vi "NewLogReader.vi"() -> ()   [LabVIEW 2011]
doc: "Reads new (11-1-2012+) style logs and displays the data in a human-understandable format."
uses:
  0-OCU/0 Typedefs/Rudder Position.ctl
  2-Think/2 Typedefs/apparent wind direction.ctl
  2-Think/2 Typedefs/apparent wind speed.ctl
  2-Think/2 Typedefs/apparent wind.ctl
  2-Think/2 Typedefs/heading.ctl
  2-Think/2 Typedefs/UTM Location.ctl
  2-Think/2 Typedefs/robot velocity.ctl
  2-Think/2 Typedefs/pitch and roll.ctl
  0-OCU/0 Typedefs/Apparent Wind Point of Sail.ctl
  0-OCU/0 Typedefs/Maps.ctl
  0-OCU/0 Typedefs/Sail Position.ctl
  2-Think/2 Typedefs/UTM Circle.ctl
  <vilib>/vision/Image Controls.llb/IMAQ Image.ctl
  2-Think/2 Classes/Waypoint/Waypoint.lvclass
panel:
  in  "Choose graph to display":T1(tab)
  out "Rudder Manual?":bool
  out "Rudder Position":T2 scale=50.0..-50.0 scale format="%#.2g"
  out "Sail Manual?":bool
  in  "OCU":enum32{"Mission Map", "Detailed Telemetry"}(tab)
  out "Heading":T3 format="%05.1f"
  out "Goodness Functions Polar Plot":picture
  in  "Plot Colors":T4={"Target"=3381759, "No Sail"=16711680, "Change"=16756736, "Pure Waypt"=35080, "Pure Wind"=16860, "Combined"=16777228}
  out "Mission Map":T5(plugin-control)
  out "Apparent Wind Direction\nPoint of Sail":T6 scale=0.0..360.0 scale format="%4d"
  in  "Font Size":i16=40
  in  "Globals":enum32{"Where Am I", "What's Around Me"}(tab)
  out "Robot Heading":T3 format="%05.1f"
  out "Robot UTM Location":T7 {"North" format="%#_10f"; "East" format="%#_8f"}
  out "Robot Velocity":T8
  out "Robot Pitch/Roll":T9 {"Roll" format="%05.1f"; "Pitch" format="%05.1f"}
  out "Robot Speed (m/s)":dbl
  out "Apparent Wind Direction":T10
  out "Apparent Wind Speed":T11
  out "Apparent Wind":T12
  in  "Map Name":T13="LPB Pool"
  out "Sail Position":T14
  out "Location":cluster{dbl[], dbl[]}[](graph)
  out "Battery Voltage":cluster{i32[], dbl[]}(graph)
  out "Velocity":cluster{i32[], dbl[]}[](graph)
  out "Headings":cluster{i32[], dbl[]}[](graph)
  out "Rudder":cluster{i32[], dbl[]}(graph)
  out "Sail":cluster{i32[], dbl[]}(graph)
  in  "Time":i32(slide) max=625 scale=0.0..42.0
  in  "stop":bool
  in  "Array":string[](array[string])=["RobotLocation", "RobotHeading", "RobotVelocity", "RobotPitch", "RobotRoll", "BatteryVoltage", "ApparentWindDirection", "ApparentWindSpeed", "Rudder", "Sail", "GoodnessFunctions", "NoSailZones", "Waypoint#", "WaypointTolerance", "WaypointCoordinates", "OverrideRudder", "OverrideSail"]
  out "Processing File....":path
  in  "Stop early":bool
  out "Percent Complete":u8(slide) scale=0.0..100.0
  # "As Measured"
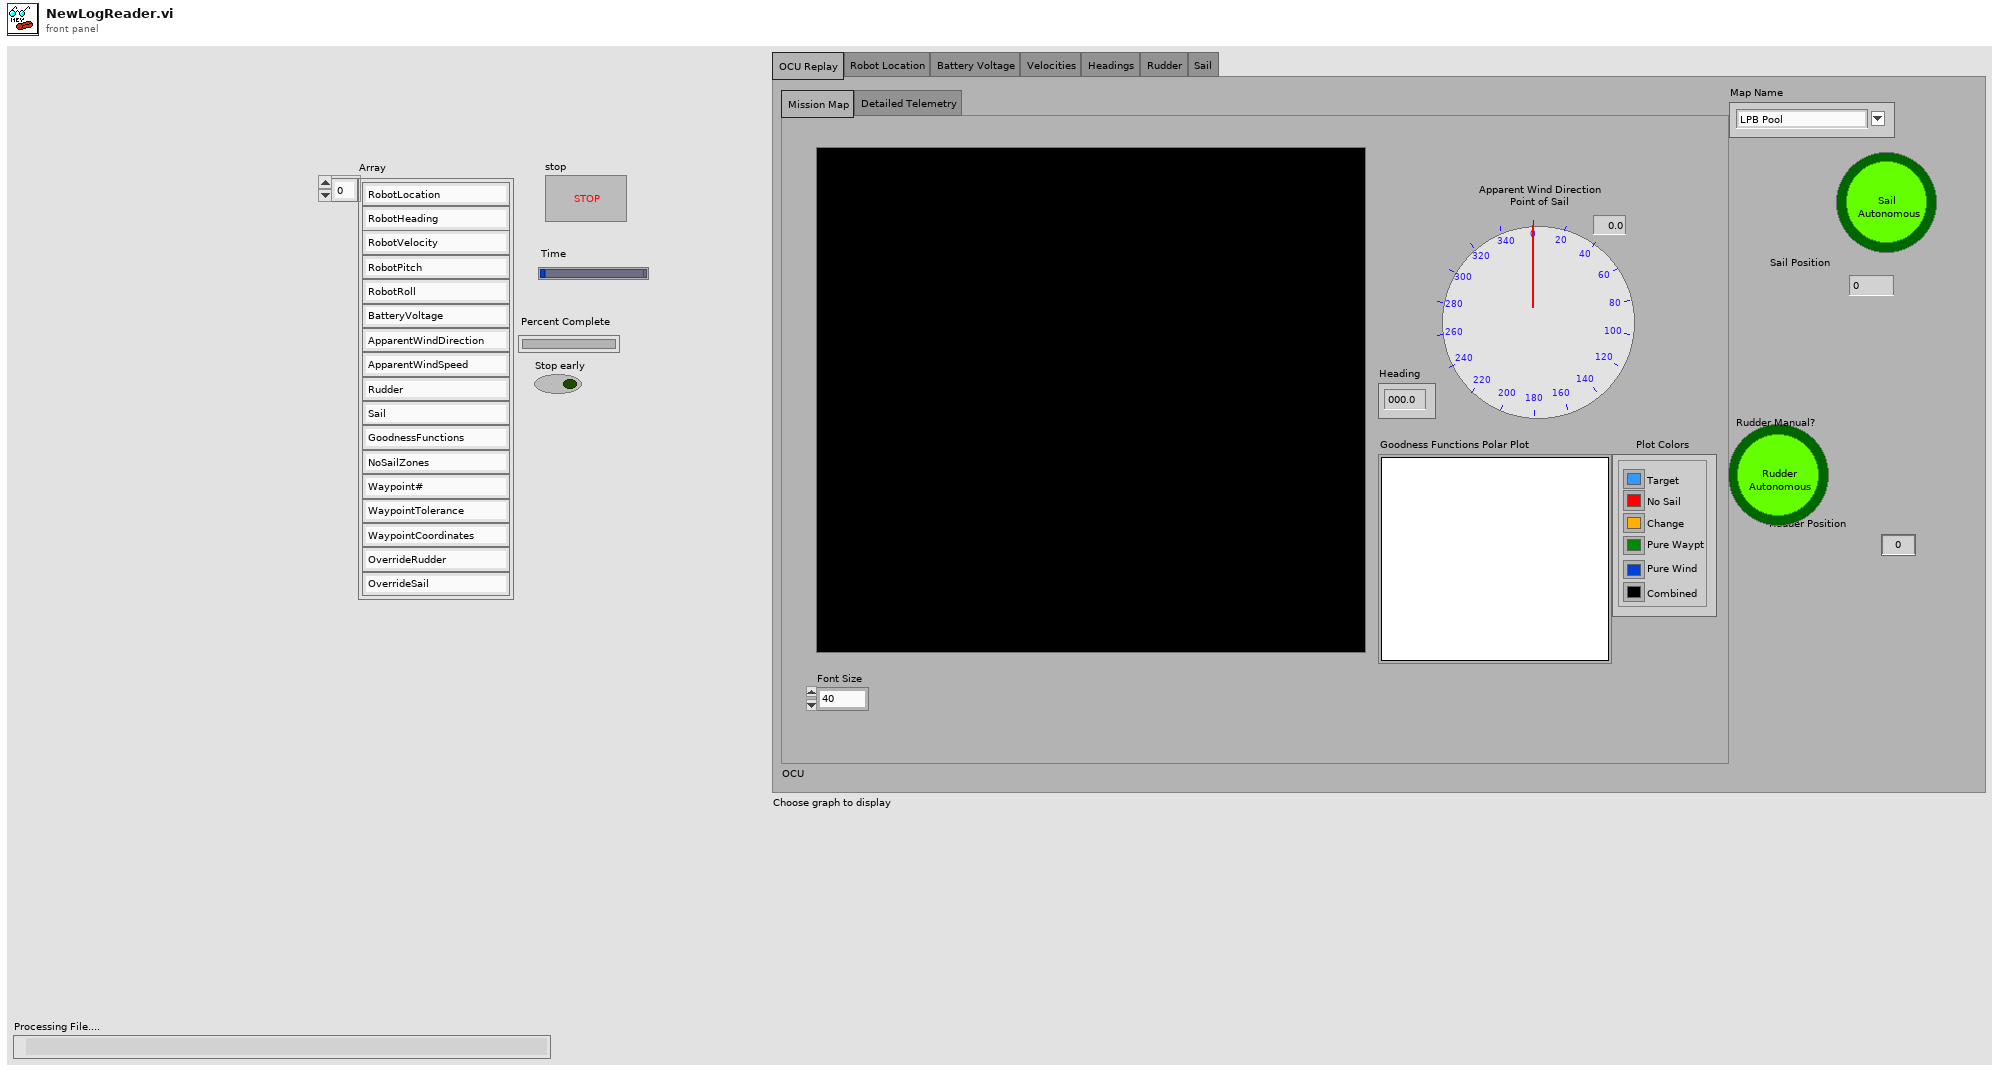
[diagram p1: front panel]
types:
  T1 = enum32{"OCU Replay", "Robot Location", "Battery Voltage", "Velocities", "Headings", "Rudder", "Sail"}
  T2 = typedef "Rudder Position.ctl" = dbl
  T3 = typedef "heading.ctl" = dbl
  T4 = cluster{"Target":u32, "No Sail":u32, "Change":u32, "Pure Waypt":u32, "Pure Wind":u32, "Combined":u32}
  T5 = typedef "IMAQ Image.ctl" = refnum<image>
  T6 = typedef "Apparent Wind Point of Sail.ctl" = dbl
  T7 = typedef "UTM Location.ctl" = cluster{"UTM Zone":dbl, "Hemisphere":enum16{"North", "South"}, "East":dbl, "North":dbl}
  T8 = typedef "robot velocity.ctl" = cluster{"East":dbl, "North":dbl}
  T9 = typedef "pitch and roll.ctl" = cluster{"Pitch":dbl, "Roll":dbl}
  T10 = typedef "apparent wind direction.ctl" = dbl
  T11 = typedef "apparent wind speed.ctl" = dbl
  T12 = typedef "apparent wind.ctl" = cluster{"Toward Fore":dbl, "Toward Starboard":dbl}
  T13 = typedef "Maps.ctl" = string
  T14 = typedef "Sail Position.ctl" = dbl
  T15 = typedef "UTM Circle.ctl" = cluster{"UTM Zone":dbl, "Hemisphere":enum16{"North", "South"}, "East":dbl, "North":dbl, "Radius":dbl}
  T16 = cluster{"RobotHeading":dbl, "RobotSpeed":dbl, "RobotPitch":dbl, "RobotRoll":dbl, "BatteryVoltage":dbl, "ApparentWindDirection":dbl, "ApparentWindSpeed":dbl, "Rudder":dbl, "Sail":dbl, "Waypoint#":dbl, "WaypointTolerance":dbl, "GoodnessFunctions":string, "OverrideRudder":bool, "OverrideSail":bool, "Global No Sail Circles":T15[], "Robot Location":T7, "WaypointCoordinates":T7}
  T17 = typedef "0-Image Descriptor.ctl" = cluster{"Upper-Left Corner Coordinates":T7, "Meters/Pixel":dbl}
  T18 = typedef "Velocity.ctl" = cluster{"East":dbl, "North":dbl}
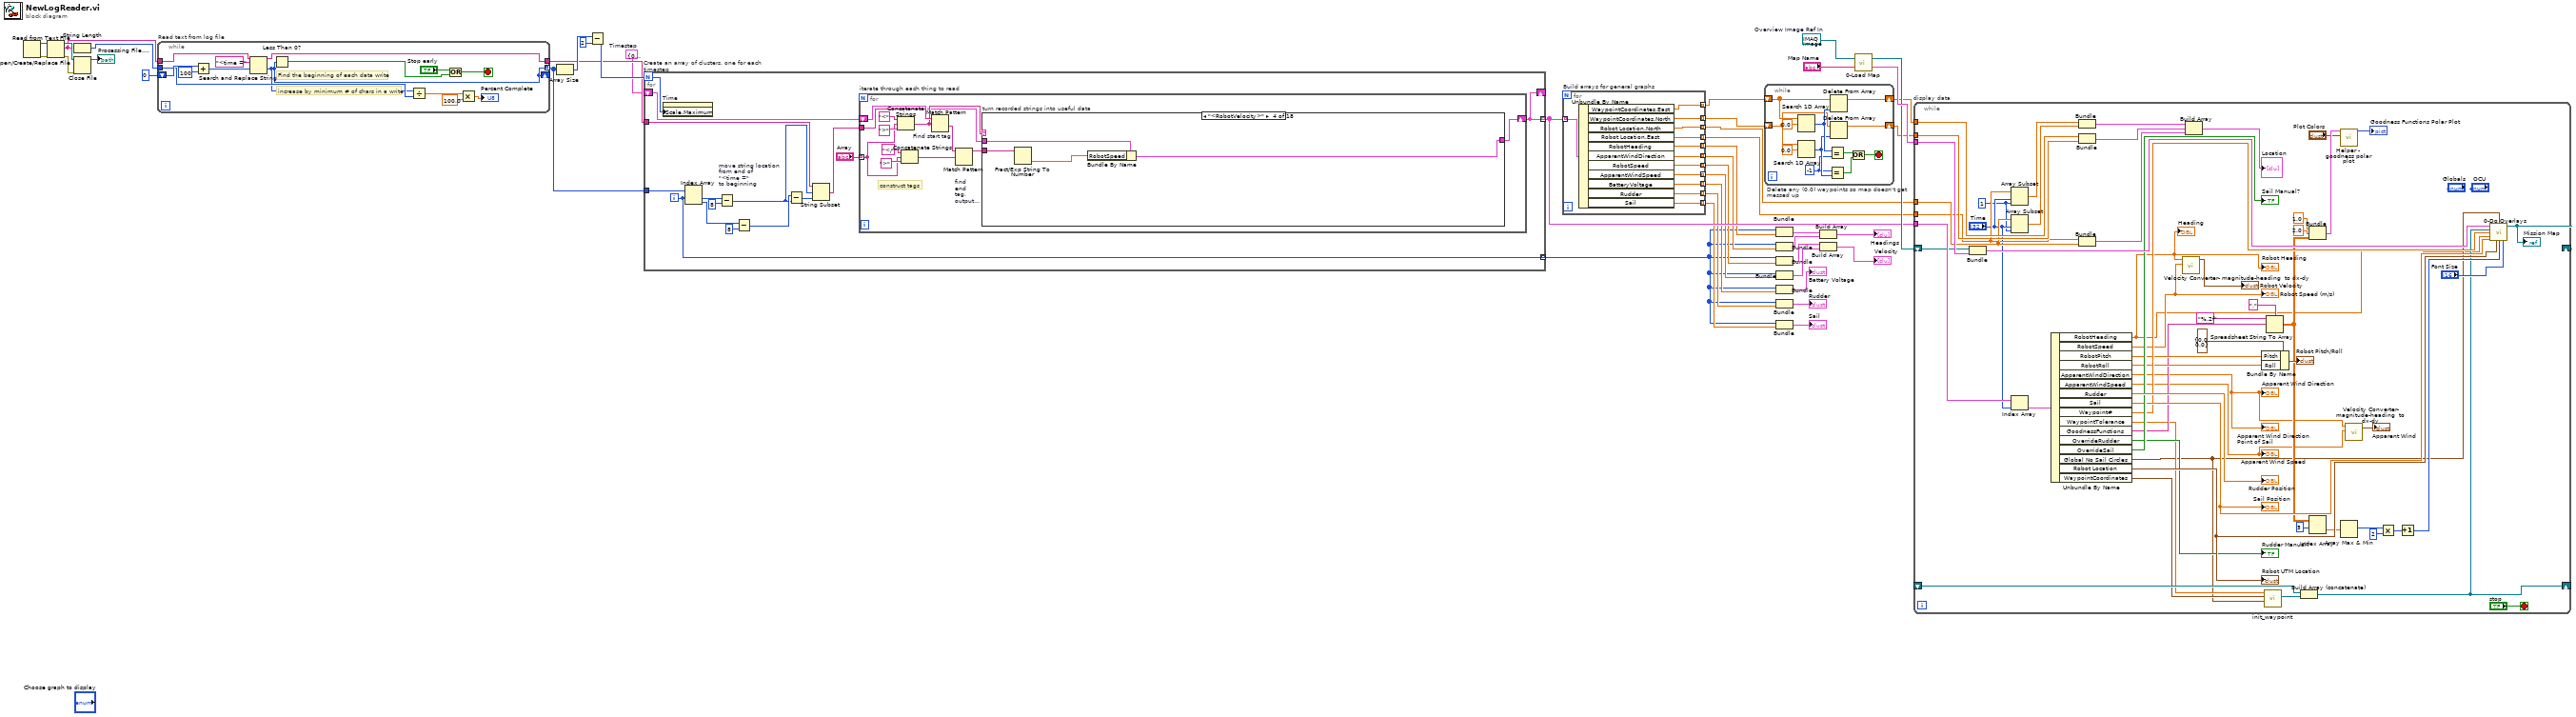
[diagram p0: block diagram]
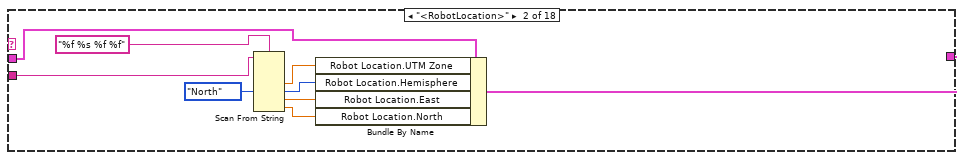
[diagram p3: hidden frame]
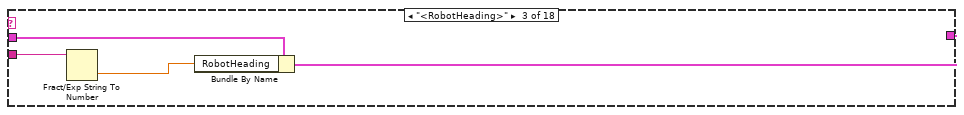
[diagram p4: hidden frame]
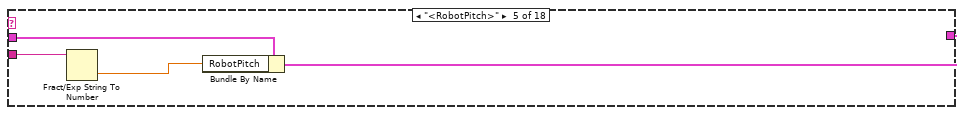
[diagram p5: hidden frame]
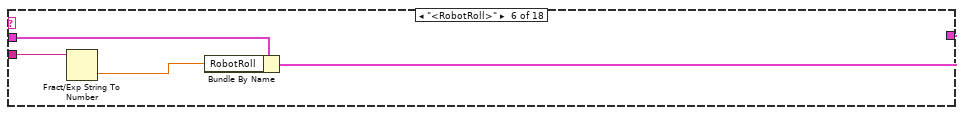
[diagram p6: hidden frame]
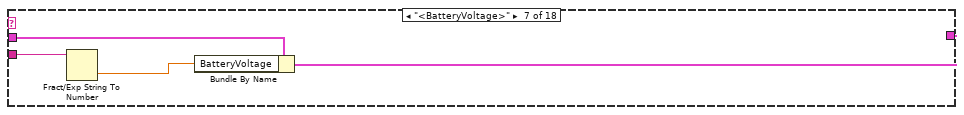
[diagram p7: hidden frame]
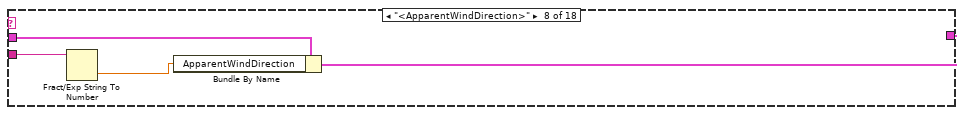
[diagram p8: hidden frame]
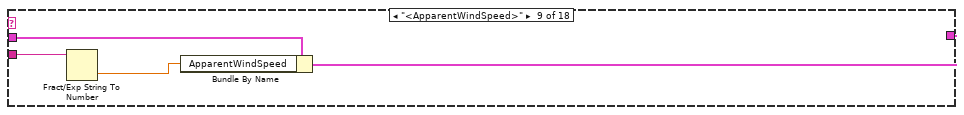
[diagram p9: hidden frame]
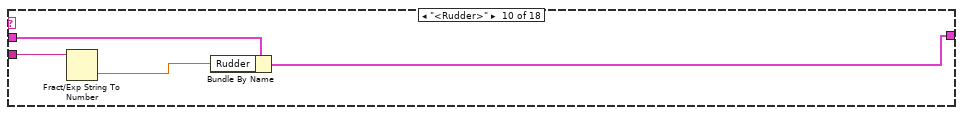
[diagram p10: hidden frame]
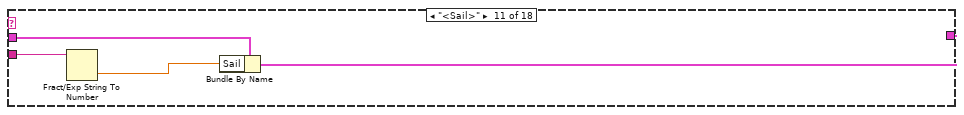
[diagram p11: hidden frame]
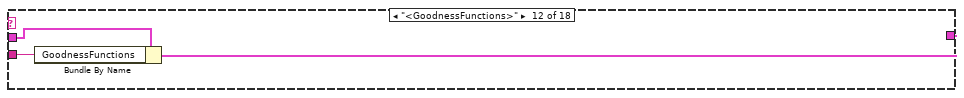
[diagram p12: hidden frame]
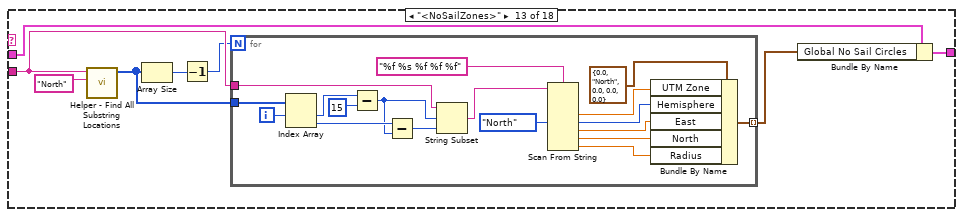
[diagram p13: hidden frame]
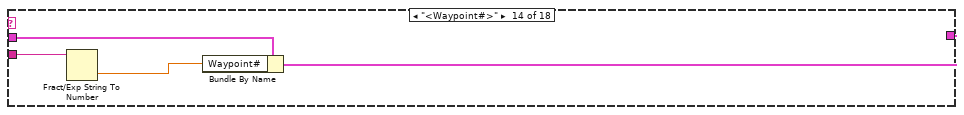
[diagram p14: hidden frame]
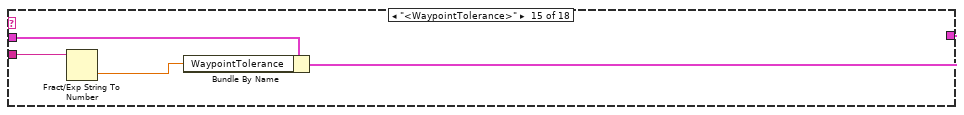
[diagram p15: hidden frame]
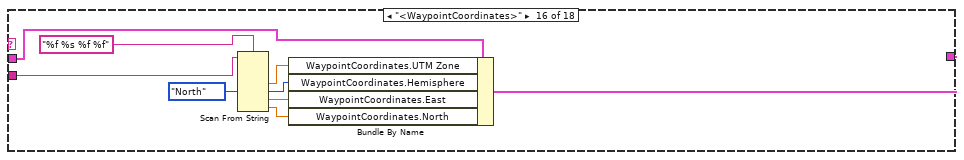
[diagram p16: hidden frame]
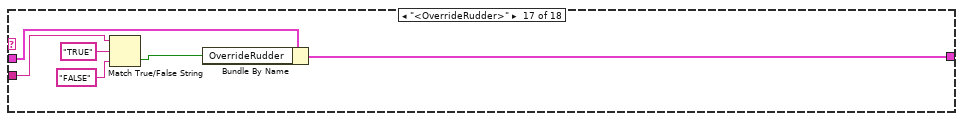
[diagram p17: hidden frame]
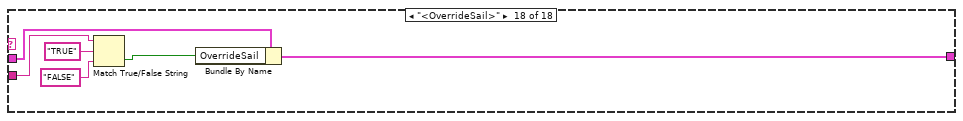
[diagram p18: hidden frame]
diagram:
  w28 = T5 refnum  # Overview Image Ref In
  w26 = T16 {"RobotHeading"=0.0, "RobotSpeed"=0.0, "RobotPitch"=0.0, "RobotRoll"=0.0, "BatteryVoltage"=0.0, "ApparentWindDirection"=0.0, "ApparentWindSpeed"=0.0, "Rudder"=0.0, "Sail"=0.0, "Waypoint#"=0.0, "WaypointTolerance"=0.0, "GoodnessFunctions"="", "OverrideRudder"=FALSE, "OverrideSail"=FALSE, "Global No Sail Circles"=[], "Robot Location"={"UTM Zone"=0.0, "Hemisphere"=enum."North", "East"=0.0, "North"=0.0}, "WaypointCoordinates"={"UTM Zone"=0.0, "Hemisphere"=enum."North", "East"=0.0, "North"=0.0}}  # Timestep
  n1 = Open/Create/Replace File() -> (refnum out=w42:refnum<file>, error out=w38:errorcluster)  [unwired: 6 in, 1 out]
  n2 = Read from Text File(file (use dialog)=w42, error in=w38) -> (refnum out=w39:refnum<file>, text=w36:string, error out=w40:errorcluster)  [unwired: 2 in, 1 out]
  n3 = String Length(string=w36) -> (length=w35:i32)
  n4 = Close File(refnum=w39, error in=w40) -> (path=→"Processing File....":path)  [unwired: 1 out]
  n5 = while "Read text from log file" {
    tunnel: w36 -> [w46]
    shift-right: [w44] -> _
    shift-left: 0 ("offset past replacement") -> [w56]
    tunnel: [w45] -> w30
    tunnel: [w44] -> w31 mode=indexing
    tunnel: w35 -> [w48]
    stop <- w54 stop-if-true
    # "increase by minimum # of chars in a write"
    # "Find the beginning of each data write"
    n6 = Add(x=w56, y=100) -> (x+y=w47:i32)
    n7 = Search and Replace String(input string=w46, search string="<time =", offset=w47) -> (result string=w45:string, offset past replacement=w44:i32)  [unwired: 5 in, 2 out]
    n8 = Less Than 0?(x=w44) -> (x < 0?=w52:bool)
    n9 = Divide(x=w44, y=w48) -> (x/y=w51:dbl)
    n10 = Or(x="Stop early", y=w52) -> (x .or. y?=w54:bool)
    n11 = Multiply(x=w51, y=100.0) -> (x*y=→"Percent Complete":dbl)
  }
  n12 = Array Size(array=w31) -> (size(s)=w34:i32)
  n13 = Subtract(x=w34, y=2) -> (x-y=w32:i32)
  n14 = for "Create an array of clusters, one for each timestep" {
    N: w32 -> [w62]
    tunnel: w31 -> [w71]
    tunnel: w30 -> [w66]
    tunnel: [w61] -> w24 mode=indexing
    shift-right: [w61] -> _
    shift-left: w26 -> [w60]
    tunnel: [w57] -> w5 mode=indexing
    i -> [w57]
    n15 = property on="Time" class="Slide (strict)"("Scale.Maximum"=w62) -> ()  [unwired: 2 in, 2 out]
    n16 = Index Array(array=w71, index #1=w57) -> (element #1=w70:i32, element #2=w67:i32)  [unwired: 1 in]
    n17 = Subtract "move string location\nfrom end of \n\"<time =\"\nto beginning"(x=w70, y=8) -> (x-y=w58:i32)
    n18 = Subtract(x=w67, y=8) -> (x-y=w59:i32)
    n19 = Subtract(x=w59, y=w58) -> (x-y=w65:i32)
    n20 = String Subset(string=w66, offset (0)=w58, length (rest)=w65) -> (substring=w64:string)
    n21 = for "iterate through each thing to read" {
      tunnel: w64 -> [w82]
      tunnel: "Array" -> [w77] mode=indexing
      shift-right: [w75] -> w61
      shift-left: w60 -> [w72]
      # "construct tags"
      n22 = Concatenate Strings("<" ("string"), w77, ">" ("string")) -> (w78:string)
      n23 = Concatenate Strings("</" ("string"), w77, ">" ("string")) -> (w79:string)
      n24 = Match Pattern "Find start tag"(string=w82, regular expression=w78) -> (after substring=w73:string)  [unwired: 1 in, 3 out]
      n25 = Match Pattern "find\nend\ntag,\noutput\nbetween\ntags"(string=w73, regular expression=w79) -> (before substring=w74:string)  [unwired: 1 in, 3 out]
      n26 = case "turn recorded strings into useful data" shown="\"<RobotVelocity>\"" w78 {
        tunnel: w74 -> [_ w87 w97 w100 w103 w108 w110 w114 w118 w122 w126 w131 w138 w160 w163 w167 w176 w182]
        tunnel: w72 -> [w84 w89 w96 w101 w104 w107 w112 w116 w120 w124 w128 w132 w137 w161 w165 w174 w179 w184]
        tunnel: [w84 w88 w94 w98 w102 w106 w111 w115 w119 w123 w127 w130 w135 w159 w164 w170 w177 w183] -> w75
        frame Default {
          # "hopefully never needs to be used"
        }
        frame "<RobotLocation>" {
          n27 = Scan From String(format string="%f %s %f %f", input string=w87, default 2=enum16{"North", "South"}."North" ("Robot Location.Hemisphere")) -> (output 1=w92:dbl, output 2=w85:enum16{"North", "South"}, output 3=w91:dbl, output 4=w90:dbl)  [unwired: 5 in, 3 out]
          n28 = Bundle By Name(cluster=w89, "Robot Location.UTM Zone"=w92, "Robot Location.Hemisphere"=w85, "Robot Location.East"=w91, "Robot Location.North"=w90) -> (w88:T16)
        }
        frame "<RobotHeading>" {
          n29 = Fract/Exp String To Number(string=w97) -> (number=w95:dbl)  [unwired: 3 in, 1 out]
          n30 = Bundle By Name(cluster=w96, "RobotHeading"=w95) -> (w94:T16)
        }
        frame "<RobotVelocity>" {
          n31 = Fract/Exp String To Number(string=w100) -> (number=w99:dbl)  [unwired: 3 in, 1 out]
          n32 = Bundle By Name(cluster=w101, "RobotSpeed"=w99) -> (w98:T16)
        }
        frame "<RobotPitch>" {
          n33 = Fract/Exp String To Number(string=w103) -> (number=w105:dbl)  [unwired: 3 in, 1 out]
          n34 = Bundle By Name(cluster=w104, "RobotPitch"=w105) -> (w102:T16)
        }
        frame "<RobotRoll>" {
          n35 = Fract/Exp String To Number(string=w108) -> (number=w109:dbl)  [unwired: 3 in, 1 out]
          n36 = Bundle By Name(cluster=w107, "RobotRoll"=w109) -> (w106:T16)
        }
        frame "<BatteryVoltage>" {
          n37 = Fract/Exp String To Number(string=w110) -> (number=w113:dbl)  [unwired: 3 in, 1 out]
          n38 = Bundle By Name(cluster=w112, "BatteryVoltage"=w113) -> (w111:T16)
        }
        frame "<ApparentWindDirection>" {
          n39 = Fract/Exp String To Number(string=w114) -> (number=w117:dbl)  [unwired: 3 in, 1 out]
          n40 = Bundle By Name(cluster=w116, "ApparentWindDirection"=w117) -> (w115:T16)
        }
        frame "<ApparentWindSpeed>" {
          n41 = Fract/Exp String To Number(string=w118) -> (number=w121:dbl)  [unwired: 3 in, 1 out]
          n42 = Bundle By Name(cluster=w120, "ApparentWindSpeed"=w121) -> (w119:T16)
        }
        frame "<Rudder>" {
          n43 = Fract/Exp String To Number(string=w122) -> (number=w125:dbl)  [unwired: 3 in, 1 out]
          n44 = Bundle By Name(cluster=w124, "Rudder"=w125) -> (w123:T16)
        }
        frame "<Sail>" {
          n45 = Fract/Exp String To Number(string=w126) -> (number=w129:dbl)  [unwired: 3 in, 1 out]
          n46 = Bundle By Name(cluster=w128, "Sail"=w129) -> (w127:T16)
        }
        frame "<GoodnessFunctions>" {
          n47 = Bundle By Name(cluster=w132, "GoodnessFunctions"=w131) -> (w130:T16)
        }
        frame "<NoSailZones>" {
          n48 = call "Helper - Find All Substring Locations.vi"("search string"="North", "input string"=w138) -> ("Locations"=w139:i32[])  [unwired: 9 in]
          n49 = Array Size(array=w139) -> (size(s)=w133:i32)
          n50 = Decrement(x=w133) -> (x-1=w134:i32)
          n51 = for {
            N: w134 -> [_]
            tunnel: w139 -> [w158]
            tunnel: w138 -> [w155]
            tunnel: [w145] -> w136 mode=indexing
            i -> [w144]
            n52 = Index Array(array=w158, index #1=w144) -> (element #1=w143:i32, element #2=w142:i32)  [unwired: 1 in]
            n53 = Subtract(x=w143, y=15) -> (x-y=w141:i32)
            n54 = Subtract(x=w142, y=w141) -> (x-y=w156:i32)
            n55 = String Subset(string=w155, offset (0)=w141, length (rest)=w156) -> (substring=w154:string)
            n56 = Scan From String(format string="%f %s %f %f %f", input string=w154, default 2=enum16{"North", "South"}."North" ("Hemisphere")) -> (output 1=w151:dbl, output 2=w149:enum16{"North", "South"}, output 3=w148:dbl, output 4=w147:dbl, output 5=w146:dbl)  [unwired: 6 in, 3 out]
            n57 = Bundle By Name(cluster=T15 {"UTM Zone"=0.0, "Hemisphere"=enum."North", "East"=0.0, "North"=0.0, "Radius"=0.0} ("UTM Location"), "UTM Zone"=w151, "Hemisphere"=w149, "East"=w148, "North"=w147, "Radius"=w146) -> (w145:T15)
          }
          n58 = Bundle By Name(cluster=w137, "Global No Sail Circles"=w136) -> (w135:T16)
        }
        frame "<Waypoint#>" {
          n59 = Fract/Exp String To Number(string=w160) -> (number=w162:dbl)  [unwired: 3 in, 1 out]
          n60 = Bundle By Name(cluster=w161, "Waypoint#"=w162) -> (w159:T16)
        }
        frame "<WaypointTolerance>" {
          n61 = Fract/Exp String To Number(string=w163) -> (number=w166:dbl)  [unwired: 3 in, 1 out]
          n62 = Bundle By Name(cluster=w165, "WaypointTolerance"=w166) -> (w164:T16)
        }
        frame "<WaypointCoordinates>" {
          n63 = Scan From String(format string="%f %s %f %f", input string=w167, default 2=enum16{"North", "South"}."North" ("WaypointCoordinates.Hemisphere")) -> (output 1=w173:dbl, output 2=w168:enum16{"North", "South"}, output 3=w172:dbl, output 4=w171:dbl)  [unwired: 5 in, 3 out]
          n64 = Bundle By Name(cluster=w174, "WaypointCoordinates.UTM Zone"=w173, "WaypointCoordinates.Hemisphere"=w168, "WaypointCoordinates.East"=w172, "WaypointCoordinates.North"=w171) -> (w170:T16)
        }
        frame "<OverrideRudder>" {
          n65 = Match True/False String(2:"FALSE" ("false string"), 3:"TRUE" ("true string"), 4:w176) -> (0:w178:bool)  [unwired: 1 out]
          n66 = Bundle By Name(cluster=w179, "OverrideRudder"=w178) -> (w177:T16)
        }
        frame "<OverrideSail>" {
          n67 = Match True/False String(2:"FALSE" ("false string"), 3:"TRUE" ("true string"), 4:w182) -> (0:w185:bool)  [unwired: 1 out]
          n68 = Bundle By Name(cluster=w184, "OverrideSail"=w185) -> (w183:T16)
        }
      }
    }
  }
  n69 = for "Build arrays for general graphs" {
    tunnel: w24 -> [w199] mode=indexing
    tunnel: [w198] -> w20 mode=indexing
    tunnel: [w197] -> w19 mode=indexing
    tunnel: [w196] -> w10 mode=indexing
    tunnel: [w195] -> w9 mode=indexing
    tunnel: [w194] -> w7 mode=indexing
    tunnel: [w193] -> w6 mode=indexing
    tunnel: [w192] -> w2 mode=indexing
    tunnel: [w191] -> w1 mode=indexing
    tunnel: [w190] -> w3 mode=indexing
    tunnel: [w189] -> w4 mode=indexing
    tunnel: [w188] -> w8 mode=indexing
    n70 = Unbundle By Name(w199) -> ("WaypointCoordinates.East"=w192:dbl, "WaypointCoordinates.North"=w191:dbl, "Robot Location.North"=w190:dbl, "Robot Location.East"=w189:dbl, "RobotHeading"=w198:dbl, "ApparentWindDirection"=w197:dbl, "RobotSpeed"=w196:dbl, "ApparentWindSpeed"=w195:dbl, "BatteryVoltage"=w188:dbl, "Rudder"=w194:dbl, "Sail"=w193:dbl)
  }
  n71 = while "Delete any (0,0) waypoints so map doesn't get messed up" {
    shift-right: [w210] -> w12
    shift-left: w2 -> [w202]
    shift-right: [w200] -> w11
    shift-left: w1 -> [w201]
    stop <- w205 stop-if-true
    w206 = -1 ("y")
    n72 = Search 1D Array(1D array=w202, element=0.0) -> (index of element=w208:i32)  [unwired: 1 in]
    n73 = Search 1D Array(1D array=w201, element=0.0) -> (index of element=w207:i32)  [unwired: 1 in]
    n74 = Equal?(x=w208, y=w206) -> (x = y?=w204:bool)
    n75 = Equal?(x=w206, y=w207) -> (x = y?=w203:bool)
    n76 = Delete From Array(array=w202, index=w208) -> (array with subset deleted=w210:dbl[])  [unwired: 1 in, 1 out]
    n77 = Delete From Array(array=w201, index=w207) -> (array with subset deleted=w200:dbl[])  [unwired: 1 in, 1 out]
    n78 = Or(x=w204, y=w203) -> (x .or. y?=w205:bool)
  }
  n79 = Bundle(w5, w20) -> (w13:cluster{i32[], dbl[]})  [unwired: 1 in]
  n80 = Bundle(w5, w19) -> (w23:cluster{i32[], dbl[]})  [unwired: 1 in]
  n81 = Bundle(w5, w10) -> (w22:cluster{i32[], dbl[]})  [unwired: 1 in]
  n82 = Bundle(w5, w9) -> (w21:cluster{i32[], dbl[]})  [unwired: 1 in]
  n83 = Bundle(w5, w8) -> (→"Battery Voltage":cluster{i32[], dbl[]})  [unwired: 1 in]
  n84 = Bundle(w5, w7) -> (→"Rudder":cluster{i32[], dbl[]})  [unwired: 1 in]
  n85 = Bundle(w5, w6) -> (→"Sail":cluster{i32[], dbl[]})  [unwired: 1 in]
  n86 = Build Array(w13, w23) -> (→"Headings":cluster{i32[], dbl[]}[])
  n87 = Build Array(w22, w21) -> (→"Velocity":cluster{i32[], dbl[]}[])
  n88 = call "0-Load Map.vi"("Map Name"="Map Name", "Image Ref In"=w28) -> ("Image Descriptor"=w27:T17, "Image Ref Out"=w25:T5)
  n89 = while "display data" {
    tunnel: w24 -> [w267]
    tunnel: w27 -> [w264]
    shift-right: [w232] -> _
    shift-left: _ -> [w236]
    shift-right: [w231] -> _
    shift-left: w25 -> [w230]
    tunnel: w12 -> [w229]
    tunnel: w11 -> [w228]
    tunnel: w3 -> [w227]
    tunnel: w4 -> [w226]
    stop <- "stop" stop-if-true
    w224 = 1 ("length")
    n90 = Bundle("Image out"=w230, "Image Descriptor"=w264) -> (w263:cluster{"Image out":T5, "Image Descriptor":T17})  [unwired: 1 in]
    n91 = Array Subset(array=w226, index="Time", length=w224) -> (w223:dbl[])
    n92 = Array Subset(array=w227, index="Time", length=w224) -> (w222:dbl[])
    n93 = Index Array(array=w267, index="Time") -> (element=w266:T16)
    n94 = Unbundle By Name(w266) -> ("RobotHeading"=w216:dbl, "RobotSpeed"=w217:dbl, "RobotPitch"=w254:dbl, "RobotRoll"=w253:dbl, "ApparentWindDirection"=w213:dbl, "ApparentWindSpeed"=w212:dbl, "Rudder"=→"Rudder Position":dbl, "Sail"=w258:dbl, "Waypoint#"=w257:dbl, "WaypointTolerance"=w235:dbl, "GoodnessFunctions"=w251:string, "OverrideRudder"=→"Rudder Manual?":bool, "OverrideSail"=→"Sail Manual?":bool, "Global No Sail Circles"=w233:T15[], "Robot Location"=w261:T7, "WaypointCoordinates"=w234:T7)
    "Apparent Wind Direction\nPoint of Sail" <- w213
    "Heading" <- w216
    "Robot Speed (m/s)" <- w217
    "Robot Heading" <- w216
    "Sail Position" <- w258
    "Robot UTM Location" <- w261
    "Apparent Wind Direction" <- w213
    "Apparent Wind Speed" <- w212
    n95 = Bundle(w223, w222) -> (w221:cluster{dbl[], dbl[]})  [unwired: 1 in]
    n96 = Bundle(w229, w228) -> (w220:cluster{dbl[], dbl[]})  [unwired: 1 in]
    n97 = Bundle(w226, w227) -> (w219:cluster{dbl[], dbl[]})  [unwired: 1 in]
    n98 = call "Velocity Converter- magnitude-heading  to dx-dy.vi"("Magnitude"=w217, "Heading"=w216) -> ("Vector Out"=→"Robot Velocity":T18)  [unwired: 9 in]
    n99 = Build Array(w221, w220, w219) -> (→"Location":cluster{dbl[], dbl[]}[])
    n100 = Bundle By Name(cluster=T9 {"Pitch"=0.0, "Roll"=0.0} ("Robot Pitch/Roll"), "Pitch"=w254, "Roll"=w253) -> (→"Robot Pitch/Roll":T9)
    n101 = call "init_waypoint.vi"("No Sail Circles"=w233, "Coords"=w234, "Tolerance (m)"=w235) -> ("Waypoint Out"=w237:refnum<class "Waypoint.lvclass">)  [unwired: 8 in]
    n102 = Spreadsheet String To Array(delimiter (Tab)=",", format string="%.2f", spreadsheet string=w251) -> (array=w240:dbl[][])  [unwired: 1 in]
    n103 = Build Array (concatenate)(w236, w237) -> (w232:refnum<class "Waypoint.lvclass">[])
    n104 = Bundle(1.0, 2.0, w240) -> (w241:cluster{dbl, dbl, dbl[][]})  [unwired: 1 in]
    n105 = Index Array(array=w240, index (row)=5 ("disabled index (col)")) -> (element=w249:dbl[])  [unwired: 1 in]
    n106 = call "Helper - goodness polar plot.vi"("Plot Colors"="Plot Colors", "Goodness Fns In"=w241) -> ("Goodness Functions Polar Plot"=→"Goodness Functions Polar Plot":picture)  [unwired: 9 in]
    n107 = Array Max & Min(array=w249) -> (max index (indices)=w248:i32)  [unwired: 3 out]
    n108 = call "Velocity Converter- magnitude-heading  to dx-dy.vi"("Magnitude"=w212, "Heading"=w213) -> ("Vector Out"=→"Apparent Wind":T18)  [unwired: 9 in]
    n109 = Multiply(x=w248, y=2) -> (x*y=w246:i32)
    n110 = Increment(x=w246) -> (x+1=w244:i32)
    n111 = call "0-Do Overlays.vi"("Image Reference\nand Descriptor"=w263, "No Sail Circles"=w233, "Waypoints"=w232, "Current Waypoint #"=w257, "Heading"=w216, "Sail Position"=w258, "Robot UTM Location"=w261, "Optimal Heading"=w244, "Font Size"="Font Size") -> ("Image out"=w231:T5)  [unwired: 6 in]
    "Mission Map" <- w231
  }
